vi "Save TS Configuration.vi"(8 "error in":errorcluster, 10 "Config File refnum in":T1, 11 "Generic Test Stand in":refnum<class "Generic Test Stand.lvclass">) -> (0 "error out":errorcluster, 2 "Config File refnum out":T1, 3 "Generic Test Stand out":refnum<class "Generic Test Stand.lvclass">)   [LabVIEW 2019, in "Generic Test Stand.lvclass"]
uses:
  Generic Test Stand.lvclass
  <vilib>/Utility/config.llb/Config Data RefNum.ctl
  Generic Test Stand.lvclass/Generic Test Stand.ctl
  <vilib>/Utility/config.llb/Write Key (String).vi
  <vilib>/Utility/config.llb/Write Key (U32).vi
  <vilib>/Utility/config.llb/NI_LVConfig.lvlib
  <vilib>/Utility/config.llb/Write Key (Double).vi
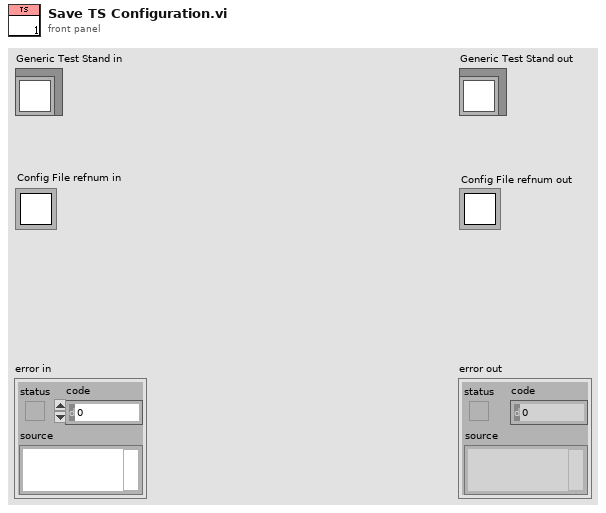
[diagram p1: front panel]
types:
  T1 = typedef "NI_LVConfig.lvlib/Config Data RefNum.ctl" = refnum<k1>
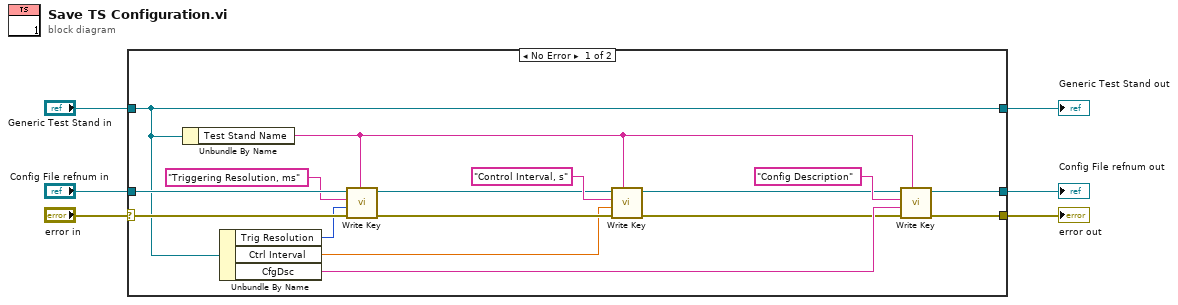
[diagram p0: block diagram]
diagram:
  n1 = case shown="No Error" "error in" {
    selector: "error in" -> [w20 w25]
    tunnel: [w19 w25] -> w5
    tunnel: [w16 w24] -> w3
    tunnel: "Generic Test Stand in" -> [w16 w24]
    tunnel: "Config File refnum in" -> [w22 w23]
    tunnel: [w18 w23] -> w1
    frame No Error {
      n2 = Unbundle By Name(w16) -> ("Test Stand Name"=w8:string)
      n3 = Unbundle By Name(w16) -> ("Trig Resolution"=w15:u32, "Ctrl Interval"=w7:dbl, "CfgDsc"=w14:string)
      n4 = call-poly <vilib>:"Write Key.vi"("section"=w8, "error in (no error)"=w20, "value"=w15, "key"="Triggering Resolution, ms", "refnum"=w22) -> ("error out"=w12:errorcluster, "refnum out"=w11:T1)  [unwired: 4 in, 1 out]
      n5 = call-poly <vilib>:"Write Key.vi"("section"=w8, "error in (no error)"=w12, "value"=w7, "key"="Control Interval, s", "refnum"=w11) -> ("error out"=w9:errorcluster, "refnum out"=w10:T1)  [unwired: 4 in, 1 out]
      n6 = call-poly <vilib>:"Write Key.vi"("section"=w8, "error in (no error)"=w9, "value"=w14, "key"="Config Description", "refnum"=w10) -> ("error out"=w19:errorcluster, "refnum out"=w18:T1)  [unwired: 4 in, 1 out]
    }
    frame Error {
    }
  }
  "error out" <- w5
  "Generic Test Stand out" <- w3
  "Config File refnum out" <- w1
